vi "Read Pressure (Raw).vi"(8 "error in (no error)":errorcluster, 11 "LPS Barometer in":refnum<class "LPS Barometric Pressure Sensor.lvclass">) -> (0 "error out":errorcluster, 2 "Raw Pressure":u32, 3 "LPS Barometer out":refnum<class "LPS Barometric Pressure Sensor.lvclass">)   [LabVIEW 2020, in "LPS Barometric Pressure Sensor.lvclass"]
uses:
  LPS Barometric Pressure Sensor.lvclass
  LINX I2C/LINX I2C.lvclass
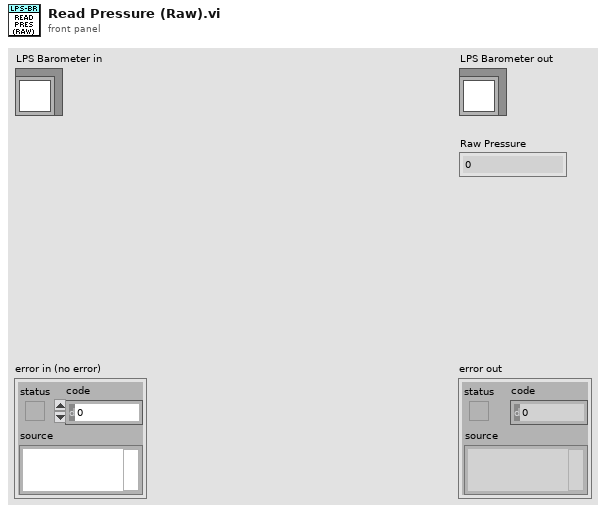
[diagram p1: front panel]
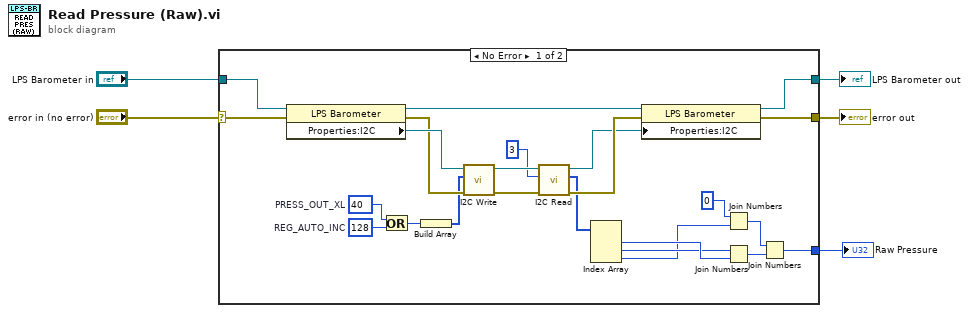
[diagram p0: block diagram]
diagram:
  n1 = case shown="No Error" "error in (no error)" {
    selector: "error in (no error)" -> [w26 w31]
    tunnel: [w18 w31] -> w4
    tunnel: [w27 w30] -> w2
    tunnel: "LPS Barometer in" -> [w29 w30]
    tunnel: [w14 _] -> w1
    frame No Error {
      w8 = u8 128  # REG_AUTO_INC
      w9 = u8 40  # PRESS_OUT_XL
      n2 = property class="LPS Barometer"(reference=w29, error in=w26) -> (reference out=w28:refnum<class "LPS Barometric Pressure Sensor.lvclass">, error out=w21:errorcluster, "Properties:I2C"=w22:refnum<class "LINX I2C.lvclass">)
      n3 = Or(x=w9, y=w8) -> (x .or. y?=w7:u8)
      n4 = Build Array(w7) -> (w6:u8[])
      n5 = call "I2C Write.vi"("error in (no error)"=w21, "Bytes to Write"=w6, "LINX I2C in"=w22) -> ("error out"=w24:errorcluster, "LINX I2C out"=w25:refnum<class "LINX I2C.lvclass">)  [unwired: 7 in]
      n6 = call-dynamic "I2C Read.vi"("error in (no error)"=w24, "# Bytes to Read"=u8 3, "LINX I2C in"=w25) -> ("error out"=w20:errorcluster, "Bytes Read"=w17:u8[], "LINX I2C out"=w19:refnum<class "LINX I2C.lvclass">)  [unwired: 6 in]
      n7 = Index Array(array=w17) -> (element #1=w13:u8, element #2=w12:u8, element #3=w11:u8)  [unwired: 3 in]
      n8 = property class="LPS Barometer"(reference=w28, error in=w20, "Properties:I2C"=w19) -> (reference out=w27:refnum<class "LPS Barometric Pressure Sensor.lvclass">, error out=w18:errorcluster)
      n9 = Join Numbers(hi=u8 0, lo=w11) -> ((hi.lo)=w16:u16)
      n10 = Join Numbers(hi=w12, lo=w13) -> ((hi.lo)=w15:u16)
      n11 = Join Numbers(hi=w16, lo=w15) -> ((hi.lo)=w14:u32)
    }
    frame Error {
    }
  }
  "error out" <- w4
  "LPS Barometer out" <- w2
  "Raw Pressure" <- w1
